vi "calculate_visible_rows_columns.vi"(8 "error in (no error)":errorcluster, 10 "actual":bool, 11 "listbox_reference":refnum<vi>) -> (0 "error out":errorcluster, 5 "visible_columns":i32, 7 "visible_rows":i32)   [LabVIEW 2015, in "lv-pagination.lvlib"]
doc: "This VI will take a given listbox reference and calculate the visible columns and rows. If pad_visible is true, it'll increment the visible rows and columns by one."
uses:
  lv-pagination.lvlib
  <vilib>/Utility/miscctls.llb/LVRowAndColumnTypeDef.ctl
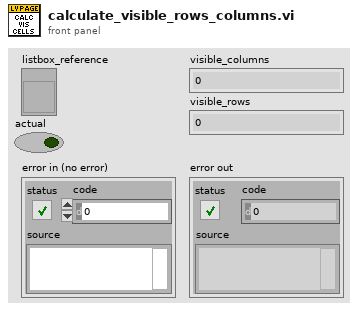
[diagram p1: front panel]
types:
  T1 = typedef "LVRowAndColumnTypeDef.ctl" = cluster{"Row":i32, "Column":i32}
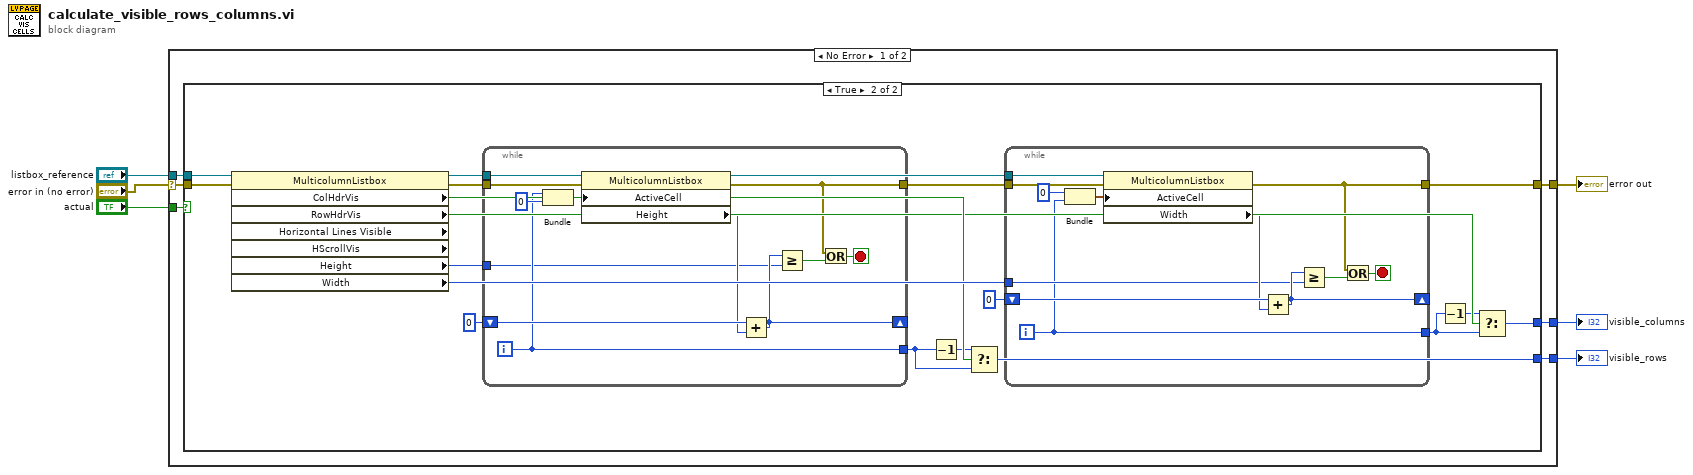
[diagram p0: block diagram]
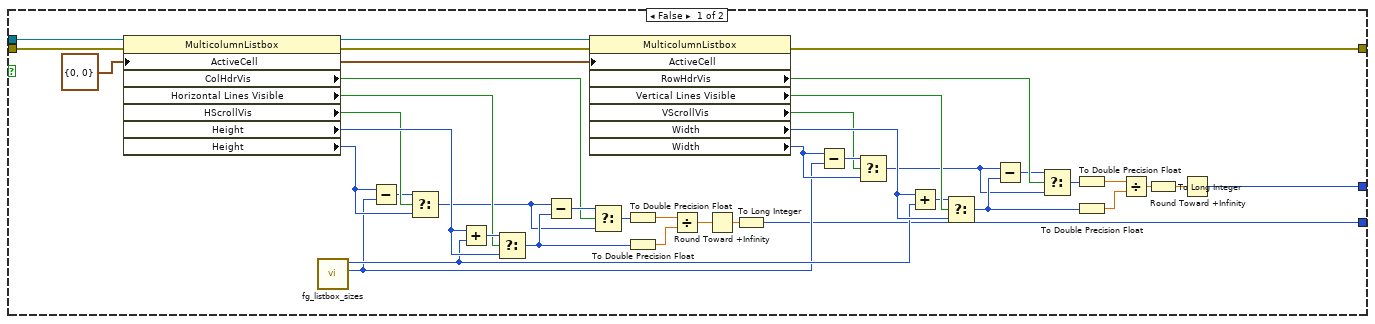
[diagram p2: hidden frame]
diagram:
  n1 = case shown="No Error" "error in (no error)" {
    selector: "error in (no error)" -> [w12 w95]
    tunnel: [w11 w95] -> w5
    tunnel: "listbox_reference" -> [w10 _]
    tunnel: [w9 _] -> w3
    tunnel: [w8 _] -> w2
    tunnel: "actual" -> [w7 _]
    frame No Error {
      n2 = case shown="True" w7 {
        tunnel: w12 -> [w52 w62]
        tunnel: [w26 w61] -> w11
        tunnel: w10 -> [w17 w63]
        tunnel: [w14 w59] -> w9
        tunnel: [w13 w56] -> w8
        frame False {
          w27 = T1 {"Row"=0, "Column"=0} ("Active Cell:Active Cell")
          n3 = property on="Property Node" class="MulticolumnListbox"(reference=w17, error in=w52, "ActiveCell"=w27) -> (reference out=w28:refnum<vi>, error out=w29:errorcluster, "ColHdrVis"=w42:bool, "Horizontal Lines Visible"=w41:bool, "HScrollVis"=w25:bool, "Height"=w45:u32, "Height"=w24:u32)
          n4 = call "fg_listbox_sizes.vi"() -> ("scrollbar_size out"=w15:u32, "line_size out"=w16:u32)  [unwired: 9 in, 1 out]
          n5 = Subtract(x=w24, y=w15) -> (x-y=w22:u32)
          n6 = Select(t=w22, s=w25, f=w24) -> (s? t:f=w23:u32)
          n7 = Add(x=w45, y=w16) -> (x+y=w44:u32)
          n8 = Select(t=w44, s=w41, f=w45) -> (s? t:f=w43:u32)
          n9 = Subtract(x=w23, y=w43) -> (x-y=w46:u32)
          n10 = property on="Property Node" class="MulticolumnListbox"(reference=w28, error in=w29, "ActiveCell"=w27) -> (error out=w26:errorcluster, "RowHdrVis"=w39:bool, "Vertical Lines Visible"=w40:bool, "VScrollVis"=w20:bool, "Width"=w36:u32, "Width"=w19:u32)  [unwired: 1 out]
          n11 = Select(t=w46, s=w42, f=w23) -> (s? t:f=w47:u32)
          n12 = To Double Precision Float(number=w47) -> (double precision float=w51:dbl)
          n13 = To Double Precision Float(number=w43) -> (double precision float=w50:dbl)
          n14 = Divide(x=w51, y=w50) -> (x/y=w49:dbl)
          n15 = Round Toward +Infinity(x=w49) -> (ceil(x): smallest int >= x=w48:dbl)
          n16 = To Long Integer(number=w48) -> (32bit integer=w14:i32)
          n17 = Subtract(x=w19, y=w15) -> (x-y=w21:u32)
          n18 = Select(t=w21, s=w20, f=w19) -> (s? t:f=w18:u32)
          n19 = Add(x=w36, y=w16) -> (x+y=w37:u32)
          n20 = Select(t=w37, s=w40, f=w36) -> (s? t:f=w38:u32)
          n21 = Subtract(x=w18, y=w38) -> (x-y=w35:u32)
          n22 = Select(t=w35, s=w39, f=w18) -> (s? t:f=w34:u32)
          n23 = To Double Precision Float(number=w34) -> (double precision float=w30:dbl)
          n24 = To Double Precision Float(number=w38) -> (double precision float=w31:dbl)
          n25 = Divide(x=w30, y=w31) -> (x/y=w32:dbl)
          n26 = Round Toward +Infinity(x=w32) -> (ceil(x): smallest int >= x=w33:dbl)
          n27 = To Long Integer(number=w33) -> (32bit integer=w13:i32)
        }
        frame True {
          n28 = property on="Property Node" class="MulticolumnListbox" props=["ColHdrVis", "RowHdrVis", "Horizontal Lines Visible", "HScrollVis", "Height", "Width"](reference=w63, error in=w62) -> (reference out=w67:refnum<vi>, error out=w69:errorcluster, "ColHdrVis"=w60:bool, "RowHdrVis"=w54:bool, "Height"=w68:u32, "Width"=w64:u32)  [unwired: 2 out]
          n29 = while {
            tunnel: w67 -> [w82]
            tunnel: w69 -> [w81]
            tunnel: [w80] -> w66
            shift-right: [w76] -> _
            shift-left: u32 0 -> [w78]
            tunnel: [w72] -> w58
            tunnel: w68 -> [w71]
            i -> [w72]
            stop <- w79 stop-if-true
            n30 = Bundle(w72, 0) -> (w74:cluster{i32, i32})  [unwired: 1 in]
            n31 = property on="Property Node" class="MulticolumnListbox"(reference=w82, error in=w81, "ActiveCell"=w74) -> (error out=w80:errorcluster, "Height"=w77:u32)  [unwired: 1 out]
            n32 = Add(x=w78, y=w77) -> (x+y=w76:u32)
            n33 = Greater Or Equal?(x=w76, y=w71) -> (x >= y?=w73:bool)
            n34 = Or(x=w80, y=w73) -> (x .or. y?=w79:bool)
          }
          n35 = Decrement(x=w58) -> (x-1=w57:i32)
          n36 = Select(t=w57, s=w60, f=w58) -> (s? t:f=w59:i32)
          n37 = while {
            tunnel: w67 -> [w94]
            tunnel: w66 -> [w93]
            tunnel: [w92] -> w61
            shift-right: [w88] -> _
            shift-left: u32 0 -> [w90]
            tunnel: [w83] -> w55
            tunnel: w64 -> [w84]
            i -> [w83]
            stop <- w91 stop-if-true
            n38 = Bundle(0, w83) -> (w86:cluster{i32, i32})  [unwired: 1 in]
            n39 = property on="Property Node" class="MulticolumnListbox"(reference=w94, error in=w93, "ActiveCell"=w86) -> (error out=w92:errorcluster, "Width"=w89:u32)  [unwired: 1 out]
            n40 = Add(x=w90, y=w89) -> (x+y=w88:u32)
            n41 = Greater Or Equal?(x=w88, y=w84) -> (x >= y?=w85:bool)
            n42 = Or(x=w92, y=w85) -> (x .or. y?=w91:bool)
          }
          n43 = Decrement(x=w55) -> (x-1=w53:i32)
          n44 = Select(t=w53, s=w54, f=w55) -> (s? t:f=w56:i32)
        }
      }
    }
    frame Error {
    }
  }
  "error out" <- w5
  "visible_rows" <- w3
  "visible_columns" <- w2
